vi "ConvertToLAB.vi"(11 "Color Box":u32(colorbox)=4390744) -> (1 "b":dbl=63.61676832347805, 2 "a":dbl=-75.6386927308898, 3 "L":dbl=88.62998039019267)   [LabVIEW 2024]
panel:
  in  "Ring":u16(ring)=5 items=["Incandescent/tungsten", "Old direct sunlight at noon", "Old daylight", "ICC profile PCS", "Mid-morning daylight", "Daylight, sRGB, Adobe-RGB", "North sky daylight", "Equal energy", "Daylight Fluorescent", "Cool fluorescent", "White Fluorescent", "Warm White Fluorescent", "Daylight Fluorescent", "Lite White Fluorescent", "Daylight fluorescent, D65 simulator", "Sylvania F40, D50 simulator", "Cool White Fluorescent", "Ultralume 50, Philips TL85", "Ultralume 40, Philips TL84", "Ultralume 30, Philips TL83"]
  in  "Table Control":string[][](table)=[["Observer", "2° (CIE 1931)", "", "", "10° (CIE 1964)", "", "", "Note"], ["Illuminant", "X2", "Y2", "Z2", "X10", "Y10", "Z10", " "], ["A", "109.850", "100.000", "35.585", "111.144", "100.000", "35.200", "Incandescent/tungsten"], ["B", "99.0927", "100.000", "85.313", "99.178;", "100.000", "84.3493", "Old direct sunlight at noon"], ["C", "98.074", "100.000", "118.232", "97.285", "100.000", "116.145", "Old daylight"], ["D50", "96.422", "100.000", "82.521", "96.720", "100.000", "81.427", "ICC profile PCS"], ["D55", "95.682", "100.000", "92.149", "95.799", "100.000", "90.926", "Mid-morning daylight"], ["D65", "95.047", "100.000", "108.883", "94.811", "100.000", "107.304", "Daylight, sRGB, Adobe-RGB"], ["D75", "94.972", "100.000", "122.638", "94.416", "100.000", "120.641", "North sky daylight"], ["E", "100.000", "100.000", "100.000", "100.000", "100.000", "100.000", "Equal energy"], ["F1", "92.834", "100.000", "103.665", "94.791", "100.000", "103.191", "Daylight Fluorescent"], ["F2", "99.187", "100.000", "67.395", "103.280", "100.000", "69.026", "Cool fluorescent"], ["F3", "103.754", "100.000", "49.861", "108.968", "100.000", "51.965", "White Fluorescent"], ["F4", "109.147", "100.000", "38.813", "114.961", "100.000", "40.963", "Warm White Fluorescent"], ["F5", "90.872", "100.000", "98.723", "93.369", "100.000", "98.636", "Daylight Fluorescent"], ["F6", "97.309", "100.000", "60.191", "102.148", "100.000", "62.074", "Lite White Fluorescent"], ["F7", "95.044", "100.000", "108.755", "95.792", "100.000", "107.687", "Daylight fluorescent, D65 simulator"], ["F8", "96.413", "100.000", "82.333", "97.115", "100.000", "81.135", "Sylvania F40, D50 simulator"], ["F9", "100.365", "100.000", "67.868", "102.116", "100.000", "67.826", "Cool White Fluorescent"], ["F10", "96.174", "100.000", "81.712", "99.001", "100.000", "83.134", "Ultralume 50, Philips TL85"], ["F11", "100.966", "100.000", "64.370", "103.866", "100.000", "65.627", "Ultralume 40, Philips TL84"], ["F12", "108.046", "100.000", "39.228", "111.428", "100.000", "40.353", "Ultralume 30, Philips TL83"]]
  out "B":u8=88
  out "G":u8=255
  out "R":u8=66
  out "Z":dbl=21.300824279367944
  out "Y":dbl=73.38283132353057
  out "X":dbl=39.76821821639694
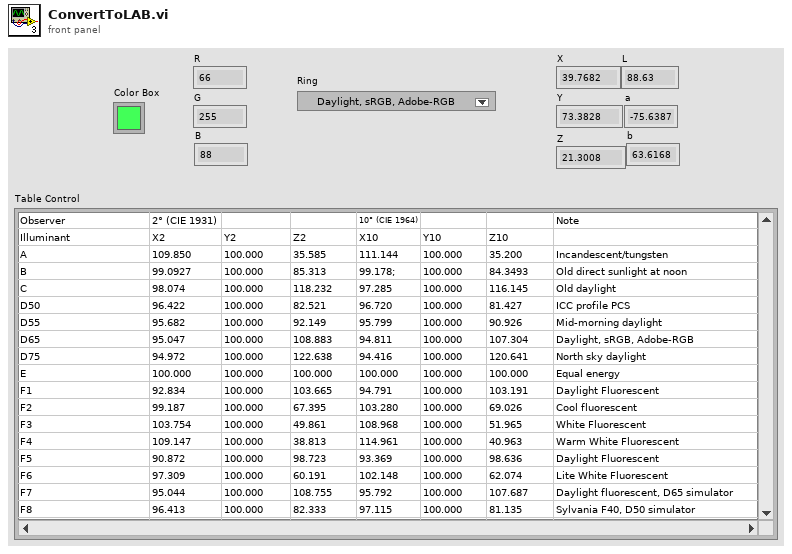
[diagram p1: front panel]
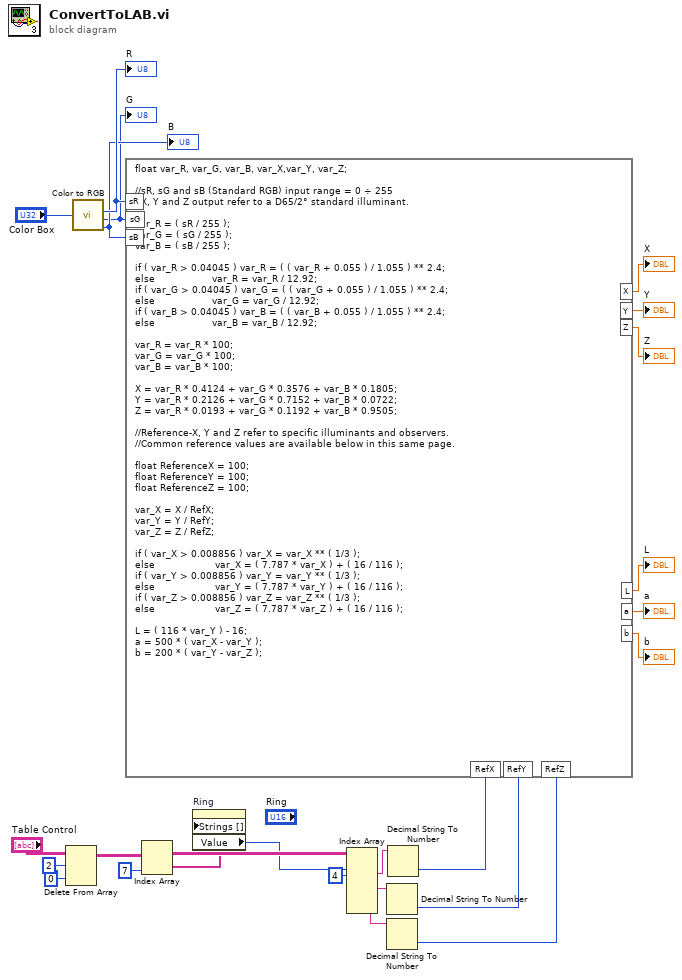
[diagram p0: block diagram]
diagram:
  n1 = Delete From Array(array="Table Control", length=2, index (row)=0) -> (array with subset deleted=w9:string[][])  [unwired: 1 in, 1 out]
  n2 = call <vilib>:"Color to RGB.vi"("Color"="Color Box") -> ("R"=w17:u8, "G"=w15:u8, "B"=w16:u8)  [unwired: 1 out]
  "R" <- w17
  "G" <- w15
  "B" <- w16
  n3 = Index Array(array=w9, index (col)=7 ("disabled index (col)")) -> (element=w8:string[])  [unwired: 1 in]
  n4 = property on="Ring" class="Ring (strict)"("Strings []"=w8) -> ("Value"=w7:u16)  [unwired: 2 in, 2 out]
  n5 = Index Array(array=w9, index (row) #1=w7, index (col) #1=4 ("index (col)")) -> (element #1=w6:string, element #2=w5:string, element #3=w4:string)  [unwired: 4 in]
  n6 = Decimal String To Number(string=w5) -> (number=w2:i32)  [unwired: 2 in, 1 out]
  n7 = Decimal String To Number(string=w4) -> (number=w1:i32)  [unwired: 2 in, 1 out]
  n8 = Decimal String To Number(string=w6) -> (number=w3:i32)  [unwired: 2 in, 1 out]
  n9 = formula code="float var_R, var_G, var_B, var_X,var_Y, var_Z;\n\n//sR, sG and sB (Standard RGB) input range = 0 ÷ 255\n//X, Y and Z output refer to a D65/2° standard illuminant.\n\nvar_R = ( sR / 255 );\nvar_G = ( sG / 255 );\nvar_B = ( sB / 255 );\n\nif ( var_R > 0.04045 ) var_R = ( ( var_R + 0.055 ) / 1.055 ) ** 2.4;\nelse                   var_R = var_R / 12.92;\nif ( var_G > 0.04045 ) var_G = ( ( var_G + 0.055 ) / 1.055 ) ** 2.4;\nelse                   var_G = var_G / 12.92;\nif ( var_B > 0.04045 ) var_B = ( ( var_B + 0.055 ) / 1.055 ) ** 2.4;\nelse                   var_B = var_B / 12.92;\n\nvar_R = var_R * 100;\nvar_G = var_G * 100;\nvar_B = var_B * 100;\n\nX = var_R * 0.4124 + var_G * 0.3576 + var_B * 0.1805;\nY = var_R * 0.2126 + var_G * 0.7152 + var_B * 0.0722;\nZ = var_R * 0.0193 + var_G * 0.1192 + var_B * 0.9505;\n\n//Reference-X, Y and Z refer to specific illuminants and observers.\n//Common reference values are available below in this same page.\n\nfloat ReferenceX = 100;\nfloat ReferenceY = 100;\nfloat ReferenceZ = 100;\n\nvar_X = X / RefX;\nvar_Y = Y / RefY;\nvar_Z = Z / RefZ;\n\nif ( var_X > 0.008856 ) var_X = var_X ** ( 1/3 );\nelse                    var_X = ( 7.787 * var_X ) + ( 16 / 116 );\nif ( var_Y > 0.008856 ) var_Y = var_Y ** ( 1/3 );\nelse                    var_Y = ( 7.787 * var_Y ) + ( 16 / 116 );\nif ( var_Z > 0.008856 ) var_Z = var_Z ** ( 1/3 );\nelse                    var_Z = ( 7.787 * var_Z ) + ( 16 / 116 );\n\nL = ( 116 * var_Y ) - 16;\na = 500 * ( var_X - var_Y );\nb = 200 * ( var_Y - var_Z );"("sR"=w17, "sG"=w15, "sB"=w16, "RefX"=w3, "RefY"=w2, "RefZ"=w1) -> ("X"=→"X":dbl, "Y"=→"Y":dbl, "Z"=→"Z":dbl, "L"=→"L":dbl, "a"=→"a":dbl, "b"=→"b":dbl)
